vi "FPGAMain.vi"() -> ()   [LabVIEW 2017]
uses:
  <vilib>/eio/EIONode/EIONode.xnode
  <vilib>/rvi/eio/common/nirviEmuTemplateMethod_errors.vi
  <vilib>/LabVIEW Targets/FPGA/RIO/nicrio_985x_controls.llb/CAN_IO_Frame Type.ctl
  <vilib>/LabVIEW Targets/FPGA/RIO/nicrio_985x_controls.llb/CAN_IO_Frame Cluster.ctl
  <vilib>/rvi/DataTransferAndStorage/Container/XNode/niFpgaContainer.xnode
  <vilib>/rvi/interface/RandomDataEmulation/nirviRandomDataFpgaReadWriteTemplate.vi
panel:
  in  "PressureSensorID":u8[](array[numeric])
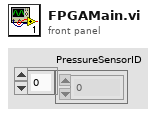
[diagram p1: front panel]
types:
  T1 = typedef "CAN_IO_Frame Cluster.ctl" = cluster{"timestamp high":u32, "timestamp low":u32, "identifier":u32, "type":T2, "info A":u8, "info B":u8, "data length":u8, "data":u8[]}
  T2 = typedef "CAN_IO_Frame Type.ctl" = enum8{"Data Frame", "Remote Frame", "(reserved)", "(reserved) ", "(reserved)  ", "(reserved)   ", "Bus Error", "Transceiver Fault"}
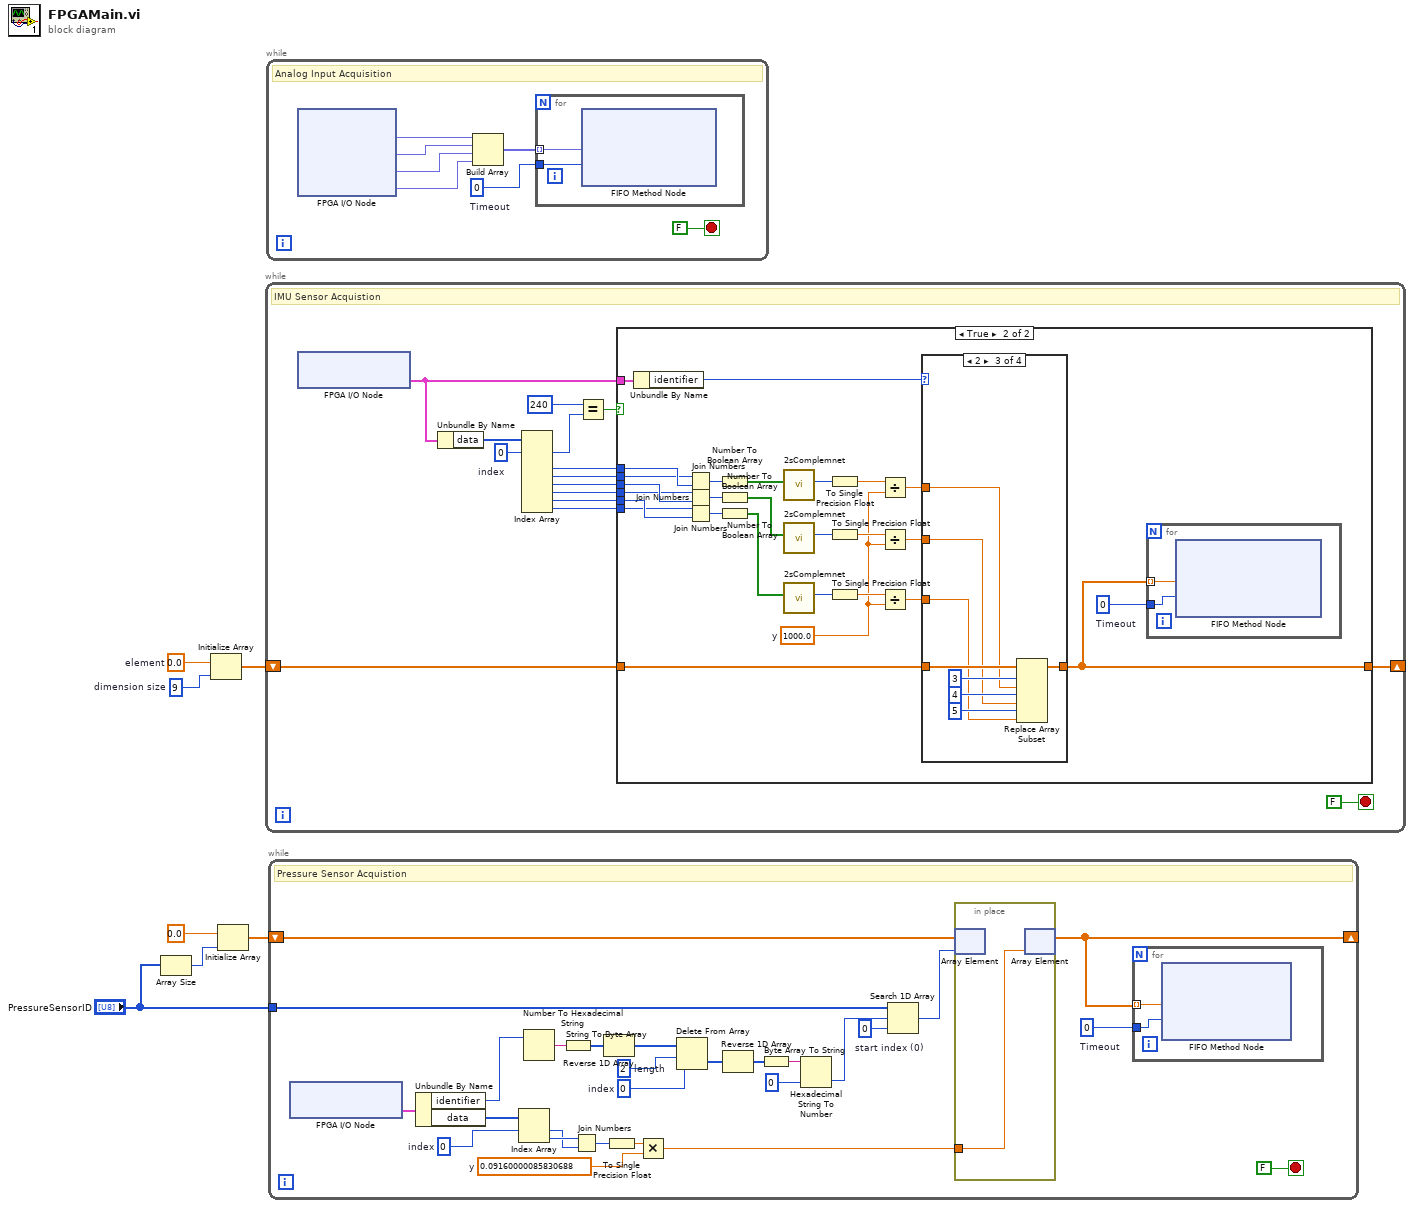
[diagram p0: block diagram]
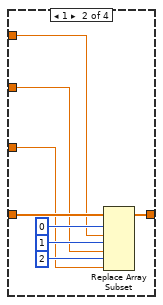
[diagram p4: hidden frame]
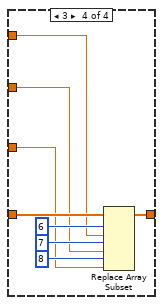
[diagram p5: hidden frame]
diagram:
  w6 = 9  # dimension size
  w7 = sgl 0.0  # element
  n1 = Array Size(array="PressureSensorID") -> (size(s)=w2:i32)
  n2 = Initialize Array "Initialize Array"(w7, w6) -> (w5:sgl[])
  n3 = Initialize Array "Initialize Array"(sgl 0.0 ("element"), w2) -> (w4:sgl[])
  n4 = while {
    shift-right: [w8] -> _
    shift-left: w5 -> [w9]
    stop <- FALSE stop-if-true
    w11 = 0  # index
    # "IMU Sensor Acquistion"
    n5 = xnode "FPGA I/O Node"() -> ("Mod2/CAN0"=w10:T1)  [unwired: 1 in, 1 out]
    n6 = Unbundle By Name(w10) -> ("data"=w13:u8[])
    n7 = Index Array "Index Array"(array=w13, index #1=w11) -> (element #1=w14:u8, element #3=w16:u8, element #4=w17:u8, element #5=w18:u8, element #6=w19:u8, element #7=w20:u8, element #8=w21:u8)  [unwired: 7 in, 1 out]
    n8 = Equal?(x=u8 240 ("y"), y=w14) -> (x = y?=w15:bool)
    n9 = case shown="True" w15 {
      tunnel: w16 -> [_ w32]
      tunnel: w17 -> [_ w31]
      tunnel: w18 -> [_ w30]
      tunnel: w19 -> [_ w29]
      tunnel: w20 -> [_ w28]
      tunnel: w21 -> [_ w27]
      tunnel: [w23 w46] -> w8
      tunnel: w10 -> [_ w50]
      tunnel: w9 -> [w23 w48]
      frame False {
      }
      frame True {
        w33 = sgl 1000.0  # y
        w47 = 0  # Timeout
        n10 = Unbundle By Name(w50) -> ("identifier"=w49:u32)
        n11 = Join Numbers(hi=w31, lo=w32) -> ((hi.lo)=w37:u16)
        n12 = Join Numbers(hi=w29, lo=w30) -> ((hi.lo)=w40:u16)
        n13 = Join Numbers(hi=w27, lo=w28) -> ((hi.lo)=w41:u16)
        n14 = Number To Boolean Array(number=w37) -> (Boolean array=w38:bool[])
        n15 = Number To Boolean Array(number=w40) -> (Boolean array=w42:bool[])
        n16 = Number To Boolean Array(number=w41) -> (Boolean array=w43:bool[])
        n17 = call "2sComplemnet.vi"("inputBitArray"=w38) -> ("outputValue"=w39:i32)  [unwired: 10 in]
        n18 = call "2sComplemnet.vi"("inputBitArray"=w42) -> ("outputValue"=w44:i32)  [unwired: 10 in]
        n19 = call "2sComplemnet.vi"("inputBitArray"=w43) -> ("outputValue"=w45:i32)  [unwired: 10 in]
        n20 = To Single Precision Float(number=w39) -> (single precision float=w36:sgl)
        n21 = To Single Precision Float(number=w44) -> (single precision float=w34:sgl)
        n22 = To Single Precision Float(number=w45) -> (single precision float=w35:sgl)
        n23 = Divide(x=w36, y=w33) -> (x/y=w26:sgl)
        n24 = Divide(x=w34, y=w33) -> (x/y=w25:sgl)
        n25 = Divide(x=w35, y=w33) -> (x/y=w24:sgl)
        n26 = case shown="2" w49 {
          tunnel: w48 -> [w53 w61 w69 w77]
          tunnel: [w53 w60 w68 w76] -> w46
          tunnel: w26 -> [_ w56 w64 w72]
          tunnel: w25 -> [_ w55 w63 w71]
          tunnel: w24 -> [_ w54 w62 w70]
          frame 0, Default {
          }
          frame 1 {
            n27 = Replace Array Subset "Replace Array Subset"(array=w61, new element #1=w56, index #1=0 ("index"), new element #2=w55, index #2=1 ("index"), new element #3=w54, index #3=2 ("index")) -> (w60:sgl[])
          }
          frame 2 {
            n28 = Replace Array Subset "Replace Array Subset"(array=w69, new element #1=w64, index #1=3 ("index"), new element #2=w63, index #2=4 ("index"), new element #3=w62, index #3=5 ("index")) -> (w68:sgl[])
          }
          frame 3 {
            n29 = Replace Array Subset "Replace Array Subset"(array=w77, new element #1=w72, index #1=6 ("index"), new element #2=w71, index #2=7 ("index"), new element #3=w70, index #3=8 ("index")) -> (w76:sgl[])
          }
        }
        n30 = for {
          tunnel: w46 -> [w52] mode=indexing
          tunnel: w47 -> [w51]
          n31 = xnode ("FIFO Method Node")("Element"=w52, "Timeout"=w51) -> ()  [unwired: 1 in, 2 out]
        }
      }
    }
  }
  n32 = while {
    stop <- FALSE stop-if-true
    w78 = 0  # Timeout
    # "Analog Input Acquisition"
    n33 = xnode "FPGA I/O Node"() -> ("Mod1/AI0"=w83:fxp<+,18,3>, "Mod1/AI1"=w82:fxp<+,18,3>, "Mod1/AI2"=w81:fxp<+,18,3>, "Mod1/AI3"=w80:fxp<+,18,3>)  [unwired: 4 in, 4 out]
    n34 = Build Array "Build Array"(w83, w82, w81, w80) -> (w79:fxp<+,18,3>[])
    n35 = for {
      tunnel: w79 -> [w86] mode=indexing
      tunnel: w78 -> [w85]
      n36 = xnode ("FIFO Method Node")("Element"=w86, "Timeout"=w85) -> ()  [unwired: 1 in, 2 out]
    }
  }
  n37 = while {
    tunnel: "PressureSensorID" -> [w91]
    shift-right: [w87] -> _
    shift-left: w4 -> [w90]
    stop <- FALSE stop-if-true
    w88 = 0  # Timeout
    w96 = 0  # index
    w97 = 2  # length
    w95 = 0  # start index (0)
    w94 = sgl 0.0916  # y
    w93 = 0  # index
    # "Pressure Sensor Acquistion"
    n38 = xnode "FPGA I/O Node"() -> ("Mod2/CAN1"=w89:T1)  [unwired: 1 in, 1 out]
    n39 = Unbundle By Name(w89) -> ("identifier"=w110:u32, "data"=w111:u8[])
    n40 = Index Array "Index Array"(array=w111, index #1=w93) -> (element #1=w99:u8, element #2=w100:u8)  [unwired: 1 in]
    n41 = Number To Hexadecimal String(2:w110) -> (0:w109:string)  [unwired: 1 in]
    n42 = String To Byte Array(string=w109) -> (unsigned byte array=w108:u8[])
    n43 = Join Numbers(hi=w100, lo=w99) -> ((hi.lo)=w101:u16)
    n44 = Reverse 1D Array(array=w108) -> (reversed array=w107:u8[])
    n45 = To Single Precision Float(number=w101) -> (single precision float=w102:sgl)
    n46 = Multiply(x=w102, y=w94) -> (x*y=w112:sgl)
    n47 = Delete From Array "Delete From Array"(array=w107, length=w97, index=w96) -> (deleted portion=w106:u8[])  [unwired: 1 out]
    n48 = Reverse 1D Array(array=w106) -> (reversed array=w105:u8[])
    n49 = Byte Array To String(unsigned byte array=w105) -> (string=w104:string)
    n50 = Hexadecimal String To Number(string=w104, default (0uL)=u8 0 ("default (0 U32)")) -> (number=w103:u8)  [unwired: 1 in, 1 out]
    n51 = Search 1D Array(1D array=w91, element=w103, start index (0)=w95) -> (index of element=w92:i32)
    n52 = in-place {
      in-place-border: w112 -> [w116]
      n53 = in-place-array #1(w90, w92) -> ()  [unwired: 1 out]
      n54 = in-place-array #1(w116) -> (w87:sgl[])  [unwired: 1 out]
    }
    n55 = for {
      tunnel: w87 -> [w115] mode=indexing
      tunnel: w88 -> [w114]
      n56 = xnode ("FIFO Method Node")("Element"=w115, "Timeout"=w114) -> ()  [unwired: 1 in, 2 out]
    }
  }
